vi "Display Info.vi"(7 "Layout ref":refnum<vi>, 8 "error in (no error)":errorcluster, 9 "Modify (F) /Add [T]":bool, 10 "Names in use":string[](array[string]), 11 "Novatech in":refnum<class "Novatech.lvclass">) -> (0 "error out":errorcluster, 1 "Names in use out":string[](array[string]), 2 "Changes Made?":bool, 3 "Novatech out":refnum<class "Novatech.lvclass">)   [LabVIEW 2013, in "Novatech.lvclass"]
uses:
  Novatech.lvclass
  TypeDefs/ColumnAppearCluster.ctl
  Novatech.lvclass/Novatech.ctl
  ColumnVIs/Column/Column.lvclass
panel:
  in  "Set Phase?":bool
  in  "Appearance in Table":T2(array[cluster])=[{"Channel Name"="0", "Columns' Appearance"=[{"Column Name"="", "Width"=30, "Bkgd"=[16448250], "Text"=[0]}, {"Column Name"="", "Width"=30, "Bkgd"=[16448250], "Text"=[0]}, {"Column Name"="", "Width"=30, "Bkgd"=[16448250], "Text"=[0]}]}, {"Channel Name"="1", "Columns' Appearance"=[{"Column Name"="", "Width"=30, "Bkgd"=[16448250], "Text"=[0]}, {"Column Name"="", "Width"=30, "Bkgd"=[16448250], "Text"=[0]}, {"Column Name"="", "Width"=30, "Bkgd"=[16448250], "Text"=[0]}]}, {"Channel Name"="2", "Columns' Appearance"=[{"Column Name"="", "Width"=30, "Bkgd"=[16448250], "Text"=[0]}, {"Column Name"="", "Width"=30, "Bkgd"=[16448250], "Text"=[0]}, {"Column Name"="", "Width"=30, "Bkgd"=[16448250], "Text"=[0]}]}, {"Channel Name"="3", "Columns' Appearance"=[{"Column Name"="", "Width"=30, "Bkgd"=[16448250], "Text"=[0]}, {"Column Name"="", "Width"=30, "Bkgd"=[16448250], "Text"=[0]}, {"Column Name"="", "Width"=30, "Bkgd"=[16448250], "Text"=[0]}]}]
  in  "Cancel":bool
  in  "Device Description":string
  in  "Name":string
  in  "Hardware Settings":T3={"PB Trigger Line"=4, "Serial Port"=""}
  in  "Done":bool
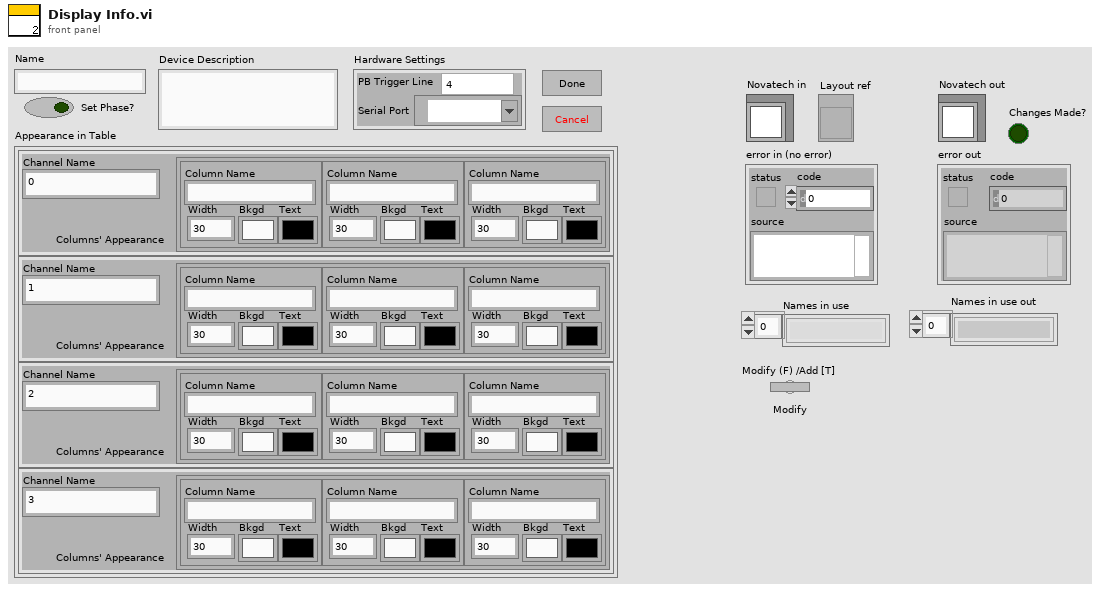
[diagram p1: front panel]
types:
  T1 = typedef "ColumnAppearCluster.ctl" = cluster{"Column Name":string, "Width":u32, "Bkgd":u32[], "Text":u32[]}
  T2 = cluster{"Channel Name":string, "Columns' Appearance":T1[]}[]
  T3 = cluster{"PB Trigger Line":u16, "Serial Port":refnum<visa-resource-name>}
  T4 = cluster{"Channel Name":bool, "Columns' Appearance":cluster{"Column Name":bool, "Width":bool, "Bkgd":bool[], "Text":bool[]}[]}[]
  T5 = cluster{"Channel Name":string, "Columns' Appearance":T1[]}
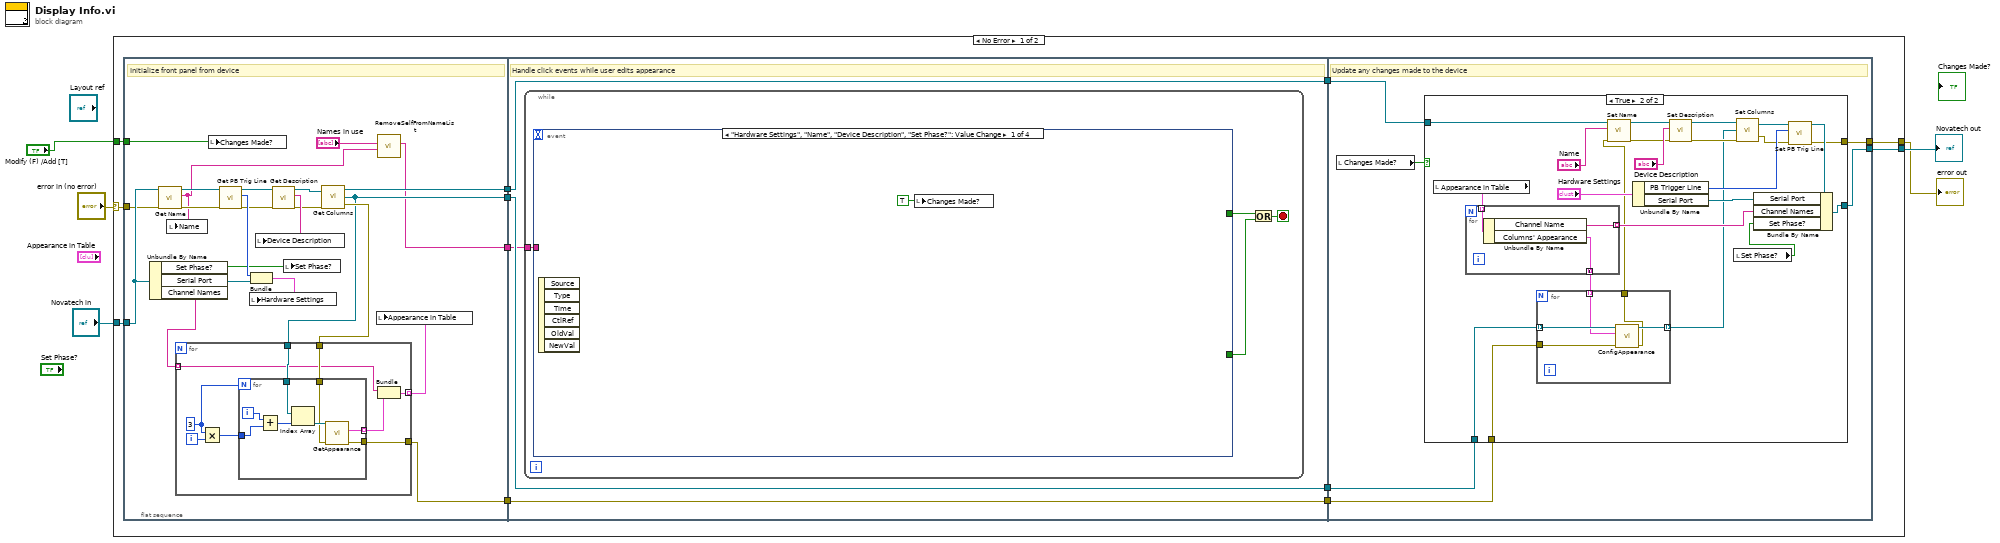
[diagram p0: block diagram]
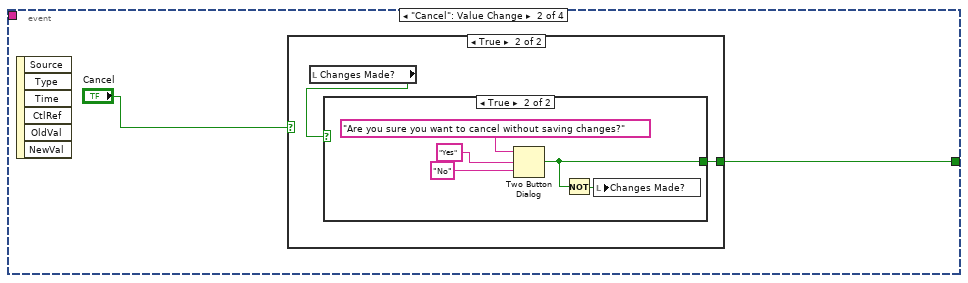
[diagram p2: hidden frame]
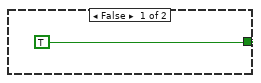
[diagram p4: hidden frame]
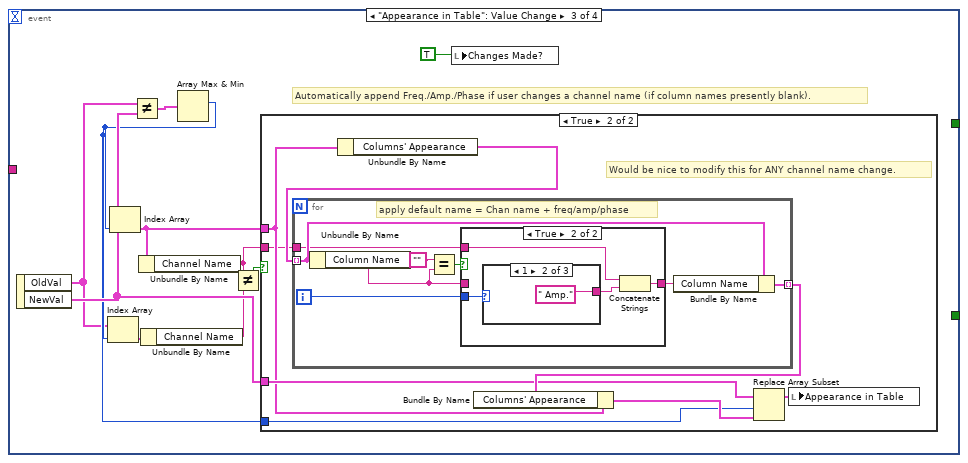
[diagram p5: hidden frame]
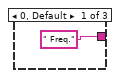
[diagram p8: hidden frame]
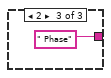
[diagram p9: hidden frame]
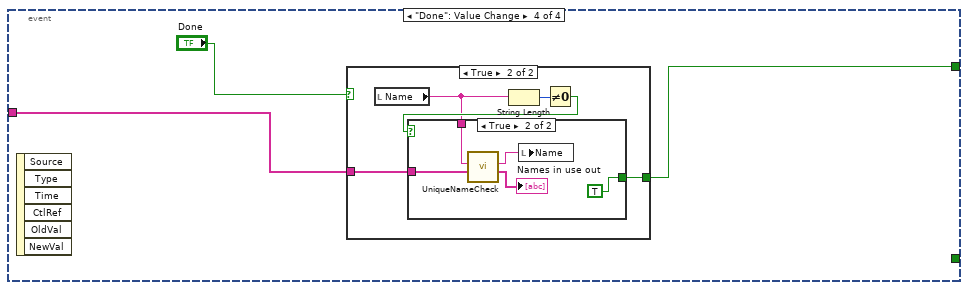
[diagram p10: hidden frame]
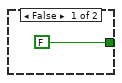
[diagram p11: hidden frame]
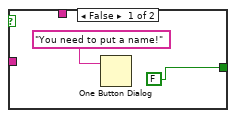
[diagram p12: hidden frame]
diagram:
  n1 = case shown="No Error" "error in (no error)" {
    selector: "error in (no error)" -> [w9 w167]
    tunnel: "Novatech in" -> [w17 w168]
    tunnel: [w16 w168] -> w4
    tunnel: [w8 w167] -> w2
    tunnel: "Modify (F) /Add [T]" -> [w7 _]
    frame No Error {
      n2 = flat-sequence {
        tunnel: w17 -> [w38]
        tunnel: [w32] -> w15
        tunnel: [w25] -> w13
        tunnel: [w24] -> w10
        tunnel: w9 -> [w23]
        tunnel: w7 -> [w22]
        tunnel: [w19] -> w6
        tunnel: w15 -> [w61]
        tunnel: [w61] -> w14
        tunnel: w13 -> [w60]
        tunnel: [w60] -> w12
        tunnel: [w59] -> w11
        tunnel: w10 -> [w59]
        tunnel: w6 -> [w58]
        tunnel: [w133] -> w16
        tunnel: w14 -> [w132]
        tunnel: w12 -> [w130]
        tunnel: w11 -> [w129]
        tunnel: [w128] -> w8
        frame #0 {
          # "Initialize front panel from device"
          n3 = Unbundle By Name(w38) -> ("Set Phase?"=w18:bool, "Serial Port"=w40:refnum<visa-resource-name>, "Channel Names"=w28:string[])
          n4 = call-dynamic "Get Name.vi"("error in (no error)"=w23, "Device in"=w38) -> ("error out"=w31:errorcluster, "Name"=w20:string, "Device out"=w39:refnum<class "Novatech.lvclass">)  [unwired: 7 in]
          n5 = local write "Name"(w20) -> ()
          n6 = local write "Changes Made?"(w22) -> ()
          n7 = call-dynamic "Get PB Trig Line.vi"("error in (no error)"=w31, "Device in"=w39) -> ("error out"=w30:errorcluster, "PB Trigger Line"=w34:u16, "Device out"=w36:refnum<class "Novatech.lvclass">)  [unwired: 7 in]
          n8 = Bundle("PB Trigger Line"=w34, "Serial Port"=w40) -> (w35:T3)  [unwired: 1 in]
          n9 = local write "Hardware Settings"(w35) -> ()
          n10 = call-dynamic "Get Description.vi"("error in (no error)"=w30, "Device in"=w36) -> ("error out"=w29:errorcluster, "Device Description"=w37:string, "Device out"=w33:refnum<class "Novatech.lvclass">)  [unwired: 7 in]
          n11 = local write "Device Description"(w37) -> ()
          n12 = local write "Set Phase?"(w18) -> ()
          n13 = call-dynamic "Get Columns.vi"("Device in"=w33, "error in (no error)"=w29) -> ("Device out"=w32:refnum<class "Novatech.lvclass">, "Columns"=w25:refnum<class "Column.lvclass">[], "error out"=w27:errorcluster)
          n14 = for {
            tunnel: w25 -> [w49]
            tunnel: w28 -> [w43] mode=indexing
            tunnel: w27 -> [w45]
            tunnel: [w42] -> w26 mode=indexing
            tunnel: [w41] -> w24
            i -> [w48]
            w46 = 3
            n15 = Multiply(x=w46, y=w48) -> (x*y=w47:i32)
            n16 = for {
              N: w46 -> [_]
              tunnel: w49 -> [w57]
              tunnel: w47 -> [w54]
              tunnel: w45 -> [w52]
              tunnel: [w51] -> w44 mode=indexing
              tunnel: [w50] -> w41
              i -> [w53]
              n17 = Add(x=w53, y=w54) -> (x+y=w56:i32)
              n18 = Index Array(array=w57, index=w56) -> (element=w55:refnum<class "Column.lvclass">)
              n19 = call "GetAppearance.vi"("error in (no error)"=w52, "Column in"=w55) -> ("error out"=w50:errorcluster, "Column Appearance"=w51:T1)  [unwired: 7 in, 1 out]
            }
            n20 = Bundle("String"=w43, w44) -> (w42:cluster{"String":string, T1[]})  [unwired: 1 in]
          }
          n21 = local write "Appearance in Table"(w26) -> ()
          n22 = call "RemoveSelfFromNameList.vi"("self Name"=w20, "Names in use"="Names in use") -> ("Reserved Names"=w19:string[])  [unwired: 9 in]
        }
        frame #1 {
          # "Handle click events while user edits appearance"
          n23 = while {
            tunnel: w58 -> [w62]
            stop <- w65 stop-if-true
            n24 = event shown="[0] \"Hardware Settings\", \"Name\", \"Device Description\", \"Set Phase?\": Value Change" {
              selector: _ -> [_ _ _ _]
              dyn-events: _ -> [_ _ _ _]
              timeout: _ -> [_ _ _ _]
              tunnel: [_ w67 _ _] -> w64
              tunnel: [_ _ _ w113] -> w63
              tunnel: w62 -> [_ _ _ w112]
              event "Hardware Settings", "Name", "Device Description", "Set Phase?": Value Change {
                n25 = event-data() -> ()  [unwired: 1 in, 6 out]
                n26 = local write "Changes Made?"(TRUE ("Changes Made?")) -> ()
              }
              event "Cancel": Value Change {
                n27 = event-data() -> ()  [unwired: 1 in, 6 out]
                n28 = case shown="True" "Cancel" {
                  selector: "Cancel" -> [w69 _]
                  tunnel: [w69 w71] -> w67
                  frame False {
                  }
                  frame True {
                    n29 = local read "Changes Made?"() -> (w70:bool)
                    n30 = case shown="True" w70 {
                      tunnel: [TRUE w74] -> w71
                      frame False {
                      }
                      frame True {
                        n31 = Two Button Dialog(message="Are you sure you want to cancel without saving changes?", 1:"No", 2:"Yes") -> (T button?=w74:bool)
                        n32 = Not(x=w74) -> (.not. x?=w73:bool)
                        n33 = local write "Changes Made?"(w73) -> ()
                      }
                    }
                  }
                }
              }
              event "Appearance in Table": Value Change {
                # "Automatically append Freq./Amp./Phase if user changes a channel name (if column names presently blank)."
                n34 = event-data() -> ("OldVal"=w83:T2, "NewVal"=w85:T2)  [unwired: 1 in]
                n35 = Not Equal?(x=w83, y=w85) -> (x != y?=w86:T4)
                n36 = Array Max & Min(array=w86) -> (max index (indices)=w84:i32)  [unwired: 3 out]
                n37 = Index Array(array=w83, index=w84) -> (element=w82:T5)
                n38 = Index Array(array=w85, index=w84) -> (element=w81:T5)
                n39 = Unbundle By Name(w81) -> ("Channel Name"=w80:string)
                n40 = Unbundle By Name(w82) -> ("Channel Name"=w79:string)
                n41 = Not Equal?(x=w80, y=w79) -> (x != y?=w78:bool)
                n42 = case shown="True" w78 {
                  tunnel: w85 -> [_ w92]
                  tunnel: w84 -> [_ w90]
                  tunnel: w81 -> [_ w89]
                  tunnel: w80 -> [_ w88]
                  frame False {
                  }
                  frame True {
                    # "Would be nice to modify this for ANY channel name change."
                    n43 = Unbundle By Name(w89) -> ("Columns' Appearance"=w95:T1[])
                    n44 = for {
                      tunnel: w95 -> [w99] mode=indexing
                      tunnel: [w100] -> w94 mode=indexing
                      tunnel: w88 -> [w98]
                      i -> [w102]
                      # "apply default name = Chan name + freq/amp/phase"
                      n45 = Unbundle By Name(w99) -> ("Column Name"=w96:string)
                      n46 = Equal?(x="", y=w96) -> (x = y?=w101:bool)
                      n47 = case shown="True" w101 {
                        tunnel: [w104 w106] -> w103
                        tunnel: w102 -> [_ w108]
                        tunnel: w98 -> [_ w105]
                        tunnel: w96 -> [w104 _]
                        frame False {
                        }
                        frame True {
                          n48 = case shown="1" w108 {
                            tunnel: [" Freq." " Amp." " Phase"] -> w107
                            frame 0, Default {
                            }
                            frame 1 {
                            }
                            frame 2 {
                            }
                          }
                          n49 = Concatenate Strings(w105, w107) -> (w106:string)
                        }
                      }
                      n50 = Bundle By Name(cluster=w99, "Column Name"=w103) -> (w100:T1)
                    }
                    n51 = Bundle By Name(cluster=w89, "Columns' Appearance"=w94) -> (w93:T5)
                    n52 = Replace Array Subset(array=w92, new element=w93, index=w90) -> (w91:T2)
                    n53 = local write "Appearance in Table"(w91) -> ()
                  }
                }
                n54 = local write "Changes Made?"(TRUE) -> ()
              }
              event "Done": Value Change {
                n55 = event-data() -> ()  [unwired: 1 in, 6 out]
                n56 = case shown="True" "Done" {
                  tunnel: [FALSE w118] -> w113
                  tunnel: w112 -> [_ w116]
                  frame False {
                  }
                  frame True {
                    n57 = local read "Name"() -> (w117:string)
                    n58 = String Length(string=w117) -> (length=w120:i32)
                    n59 = Not Equal To 0?(x=w120) -> (x != 0?=w119:bool)
                    n60 = case shown="True" w119 {
                      tunnel: [FALSE TRUE] -> w118
                      tunnel: w117 -> [_ w126]
                      tunnel: w116 -> [_ w124]
                      frame False {
                        n61 = One Button Dialog(message="You need to put a name!") -> ()  [unwired: 1 in, 1 out]
                      }
                      frame True {
                        n62 = call "UniqueNameCheck.vi"("Names in use"=w124, "Device Name"=w126) -> ("Names in use out"=→"Names in use out":string[], "Unique name"=w125:string)  [unwired: 8 in]
                        n63 = local write "Name"(w125) -> ()
                      }
                    }
                  }
                }
              }
            }
            n64 = Or(x=w63, y=w64) -> (x .or. y?=w65:bool)
          }
        }
        frame #2 {
          # "Update any changes made to the device"
          n65 = local read "Changes Made?"() -> (w131:bool)
          n66 = case shown="True" w131 {
            tunnel: [w135 w158] -> w133
            tunnel: w132 -> [w135 w153]
            tunnel: w130 -> [_ w142]
            tunnel: w129 -> [w134 w140]
            tunnel: [w134 w138] -> w128
            frame False {
            }
            frame True {
              n67 = local read "Appearance in Table"() -> (w143:T2)
              n68 = for {
                tunnel: [w166] -> w157 mode=indexing
                tunnel: w143 -> [w165] mode=indexing
                tunnel: [w164] -> w141 mode=concatenating
                n69 = Unbundle By Name(w165) -> ("Channel Name"=w166:string, "Columns' Appearance"=w164:T1[])
              }
              n70 = for {
                tunnel: w142 -> [w163] mode=indexing
                tunnel: w141 -> [w162] mode=indexing
                tunnel: w140 -> [w161]
                tunnel: [w160] -> w139 mode=indexing
                tunnel: [w159] -> w137
                n71 = call "ConfigAppearance.vi"("error in (no error)"=w161, "Column Appearance"=w162, "Column in"=w163) -> ("error out"=w159:errorcluster, "Column out"=w160:refnum<class "Column.lvclass">)  [unwired: 7 in]
              }
              n72 = call-dynamic "Set Name.vi"("error in (no error)"=w137, "Name"="Name", "Device in"=w153) -> ("error out"=w145:errorcluster, "Device out"=w155:refnum<class "Novatech.lvclass">)  [unwired: 7 in]
              n73 = Unbundle By Name("Hardware Settings") -> ("PB Trigger Line"=w148:u16, "Serial Port"=w150:refnum<visa-resource-name>)
              n74 = call-dynamic "Set Description.vi"("error in (no error)"=w145, "Device Description"="Device Description", "Device in"=w155) -> ("error out"=w144:errorcluster, "Device out"=w154:refnum<class "Novatech.lvclass">)  [unwired: 7 in]
              n75 = local read "Set Phase?"() -> (w136:bool)
              n76 = call-dynamic "Set Columns.vi"("error in (no error)"=w144, "Columns in"=w139, "Novatech in"=w154) -> ("error out"=w146:errorcluster, "Novatech out"=w147:refnum<class "Novatech.lvclass">)  [unwired: 1 in]
              n77 = call-dynamic "Set PB Trig Line.vi"("error in (no error)"=w146, "PB Trigger Line"=w148, "Device in"=w147) -> ("error out"=w138:errorcluster, "Device out"=w149:refnum<class "Novatech.lvclass">)  [unwired: 7 in]
              n78 = Bundle By Name(cluster=w149, "Serial Port"=w150, "Channel Names"=w157, "Set Phase?"=w136) -> (w158:refnum<class "Novatech.lvclass">)
            }
          }
        }
      }
    }
    frame Error {
    }
  }
  "error out" <- w2
  "Novatech out" <- w4
